vi "Test Matrix Type.vi"   [LabVIEW 2014, in "NI_AALPro.lvlib"]
doc: "Tests whether<B> Input Matrix</B> is a matrix of special type. Wire data to the <B>Input Matrix</B> input to determine the polymorphic instance to use or manually select the instance."
uses:
  NI_AALPro.lvlib
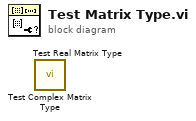
[diagram p0: block diagram]
diagram:
  n1 = call "Test Complex Matrix Type.vi"() -> ()  [unwired: 10 in, 2 out]
  n2 = call "Test Real Matrix Type.vi"() -> ()  [unwired: 10 in, 2 out]
